vi "LED and Button.vi"() -> ()   [LabVIEW 2021]
panel:
  out "Led":bool
  in  "Boton":bool
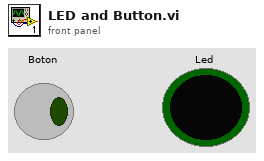
[diagram p1: front panel]
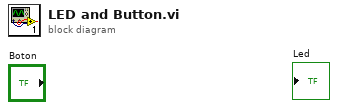
[diagram p0: block diagram]
diagram:
